vi "Contaseña.vi"(2 "spreadsheet string":string, 3 "AddContraseña":string, 4 "addUsuario":string) -> (0 "result":bool, 1 "array":string[][](array[string]))   [LabVIEW 2017]
panel:
  out "Numeros":bool
  out "Minusculas":bool
  out "Mayusculas":bool
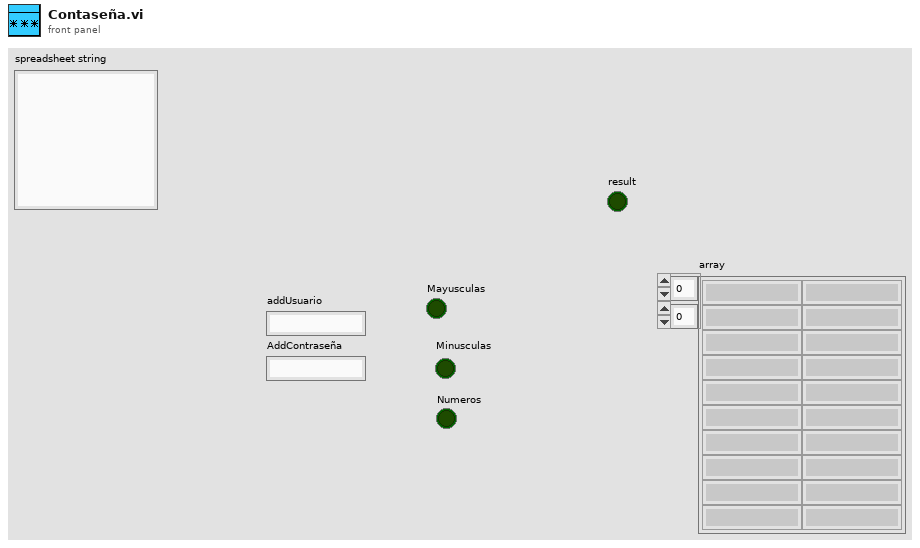
[diagram p1: front panel]
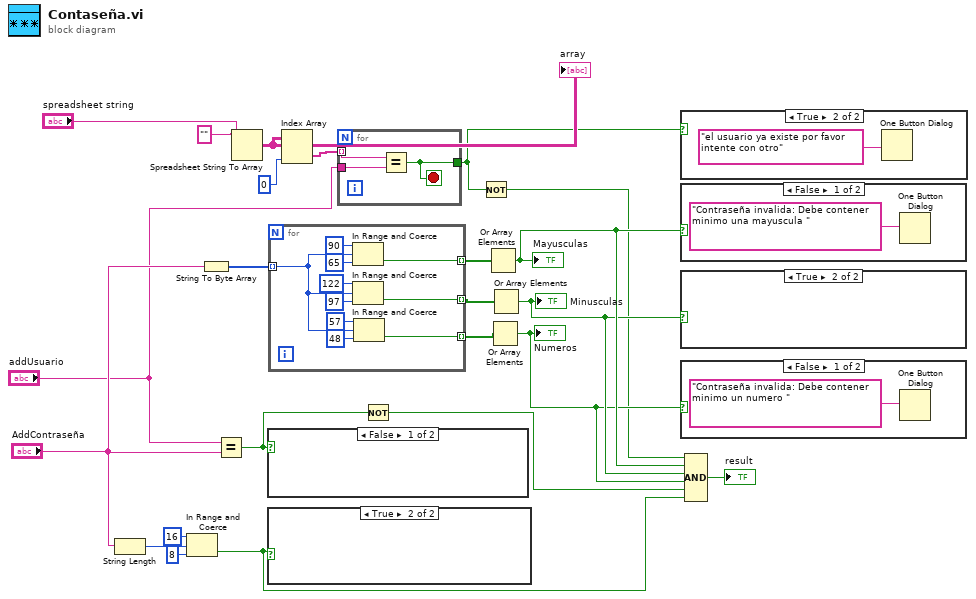
[diagram p0: block diagram]
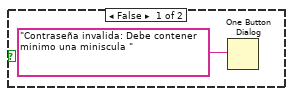
[diagram p4: hidden frame]
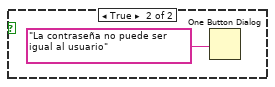
[diagram p6: hidden frame]
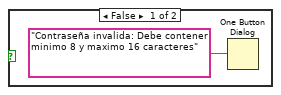
[diagram p7: hidden frame]
diagram:
  w5 = "" ("format string")
  n1 = String Length(string="AddContraseña") -> (length=w19:i32)
  n2 = In Range and Coerce(upper limit=16, x=w19, lower limit=8) -> (In Range?=w11:bool)  [unwired: 1 out]
  n3 = String To Byte Array(string="AddContraseña") -> (unsigned byte array=w23:u8[])
  n4 = Equal?(x="addUsuario", y="AddContraseña") -> (x = y?=w12:bool)
  n5 = Spreadsheet String To Array(format string=w5, spreadsheet string="spreadsheet string", array type (2D Dbl)=w5) -> (array=w6:string[][])  [unwired: 1 in]
  "array" <- w6
  n6 = case shown="False" w12 {
    frame False {
    }
    frame True {
      n7 = One Button Dialog(message="La contraseña no puede ser igual al usuario") -> ()  [unwired: 1 in, 1 out]
    }
  }
  n8 = case shown="True" w11 {
    frame False {
      n9 = One Button Dialog(message="Contraseña invalida: Debe contener minimo 8 y maximo 16 caracteres") -> ()  [unwired: 1 in, 1 out]
    }
    frame True {
    }
  }
  n10 = for {
    tunnel: w23 -> [w35] mode=indexing
    tunnel: [w32] -> w22 mode=indexing
    tunnel: [w31] -> w20 mode=indexing
    tunnel: [w30] -> w21 mode=indexing
    n11 = In Range and Coerce(upper limit=u8 90, x=w35, lower limit=u8 65) -> (In Range?=w32:bool)  [unwired: 1 out]
    n12 = In Range and Coerce(upper limit=u8 122, x=w35, lower limit=u8 97) -> (In Range?=w31:bool)  [unwired: 1 out]
    n13 = In Range and Coerce(upper limit=u8 57, x=w35, lower limit=u8 48) -> (In Range?=w30:bool)  [unwired: 1 out]
  }
  n14 = Index Array(array=w6, index (col)=0 ("disabled index (col)")) -> (element=w8:string[])  [unwired: 1 in]
  n15 = for {
    tunnel: "addUsuario" -> [w38]
    tunnel: w8 -> [w37] mode=indexing
    tunnel: [w36] -> w2
    stop <- w36 stop-if-true
    n16 = Equal?(x=w37, y=w38) -> (x = y?=w36:bool)
  }
  n17 = Not(x=w12) -> (.not. x?=w9:bool)
  n18 = Not(x=w2) -> (.not. x?=w3:bool)
  n19 = Or Array Elements(Boolean array=w22) -> (logical OR=w15:bool)
  "Mayusculas" <- w15
  n20 = Or Array Elements(Boolean array=w21) -> (logical OR=w13:bool)
  "Numeros" <- w13
  n21 = Or Array Elements(Boolean array=w20) -> (logical OR=w14:bool)
  "Minusculas" <- w14
  n22 = case shown="True" w2 {
    frame False {
    }
    frame True {
      n23 = One Button Dialog(message="el usuario ya existe por favor intente con otro") -> ()  [unwired: 1 in, 1 out]
    }
  }
  n24 = case shown="False" w15 {
    frame False {
      n25 = One Button Dialog(message="Contraseña invalida: Debe contener minimo una mayuscula ") -> ()  [unwired: 1 in, 1 out]
    }
    frame True {
    }
  }
  n26 = case shown="True" w14 {
    frame False {
      n27 = One Button Dialog(message="Contraseña invalida: Debe contener minimo una miniscula ") -> ()  [unwired: 1 in, 1 out]
    }
    frame True {
    }
  }
  n28 = case shown="False" w13 {
    frame False {
      n29 = One Button Dialog(message="Contraseña invalida: Debe contener minimo un numero ") -> ()  [unwired: 1 in, 1 out]
    }
    frame True {
    }
  }
  n30 = Compound Arithmetic op=AND(w3, w15, w14, w13, w9, w11) -> (→"result":bool)
